vi "ultratest.vi"   [LabVIEW 2010, in "Test1.lvrbt"]
uses:
  Test1.lvrbt
  <vilib>/NXT/Block Support/NXT_InputPort.ctl
  <vilib>/NXT/Subs/MotorOutput.ctl
  <vilib>/NXT/Dual Mode Library/Sensors/Sonar_cm.vi
  <vilib>/NXT/Dual Mode Library/Motors/MotorOn.vi
types:
  T1 = typedef "NXT_InputPort.ctl" = u8
  T2 = typedef "MotorOutput.ctl" = u8
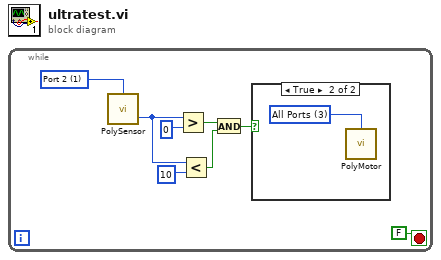
[diagram p0: block diagram]
diagram:
  n1 = while {
    stop <- FALSE stop-if-true
    w1 = T1 1 items=["Port 1", "Port 2", "Port 3", "Port 4"] ("Port (Port 4)")
    n2 = call-poly <vilib>:"PolySensor.vi"("Port (Port 4)"=w1) -> ("Distance (cm)"=w7:i16)  [unwired: 2 in, 1 out]
    n3 = Greater?(x=w7, y=i16 0) -> (0:w4:bool)
    n4 = Less?(x=w7, y=i16 10) -> (x < y?=w3:bool)
    n5 = And(x=w4, y=w3) -> (x .and. y?=w2:bool)
    n6 = case shown="True" w2 {
      frame False {
      }
      frame True {
        w9 = T2 3 items=["Port A"=0, "Port B"=1, "Port C"=2, "Ports A & B"=4, "Ports A & C"=5, "Ports B & C"=6, "All Ports"=3] ("Output Port (All Ports)")
        n7 = call-poly <vilib>:"PolyMotor.vi"("Output Port (All Ports)"=w9) -> ()  [unwired: 3 in, 1 out]
      }
    }
  }
